vi "Finish Stream.vi"(8 "error in (no error)":errorcluster, 10 "New Mode":T1, 11 "Application in":refnum<class "Application.lvclass">) -> (0 "error out":errorcluster, 3 "Application out":refnum<class "Application.lvclass">)   [LabVIEW 2018, in "Application.lvlib" / "Application.lvclass"]
uses:
  Application.lvclass
  Mode.ctl
  Application.lvclass/Application.ctl
  Hardware/Synchronization Device Messages/Set Streaming Msg/Set Streaming Msg.lvclass/Set Streaming Msg.ctl
  <vilib>/ActorFramework/Message Enqueuer/Message Enqueuer.lvclass/Message Enqueuer.ctl
  Hardware/Tiff Writer/Tiff Writer Messages/Save Tiff Msg/Save Tiff Msg.lvclass/Save Tiff Msg.ctl
  <vilib>/ActorFramework/Message Enqueuer/Enqueue.vi
  Hardware/Synchronization Device Messages/Set Streaming Msg/Set Streaming Msg.lvclass
  C:/Program Files/National Instruments/LabVIEW 2018/vi.lib/ActorFramework/Message/Message.lvclass
  Hardware/Camera Messages/Finish Stream Msg/Finish Stream Msg.lvclass
  Hardware/Tiff Writer/Tiff Writer Messages/Save Tiff Msg/Save Tiff Msg.lvclass
  Resources/GLOBAL/GLOBAL Time-critical.vi
  <vilib>/ActorFramework/Message Priority Queue/Priority Enqueue.vi
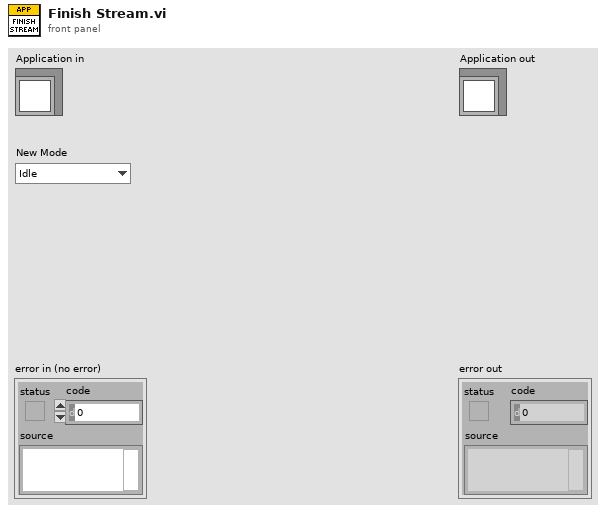
[diagram p1: front panel]
types:
  T1 = typedef "Mode.ctl" = enum16{"Idle", "Cancel", "Live", "Stream", "Autofocus", "Z-Stack"}
  T2 = typedef "Camera Settings.ctl" = cluster{"Exposure Time (ms)":dbl, "Binning":enum16{"1x1", "2x2", "4x4"}, "Scan Mode":i32, "Frames to Acquire":dbl, "Pixel Correction":bool, "Frames to Skip":u32, "File Path":path, "Duty cycle":dbl, "ALEX":bool, "Shutter Enable":bool[], "Timelapse Interval (s)":u32, "fluidics trigger frame":u16}
  T3 = cluster{"Number of Frames":u32, "Image Width (px)":u32, "Image Height (px)":u32, "Pixel Size (nm)":dbl, "Exposure Time (ms)":dbl, "Frame Time (ms)":dbl, "Number of Channels":u32, "Camera Type":enum16{"<unknown>", "Evolve 512", "Orca-Flash 4.0 V2"}, "Bit Depth":u32, "Image Description":string}
  T4 = typedef "Physical Camera Assignment.ctl" = cluster{"Channel Name":string, "Camera Type":T5, "Serial Number":string, "Flip Vertically":bool, "Flip Horizontally":bool, "photonsPerCount":dbl, "wavelength":i16}
  T5 = typedef "Camera Type.ctl" = enum16{"Hamamatsu"}
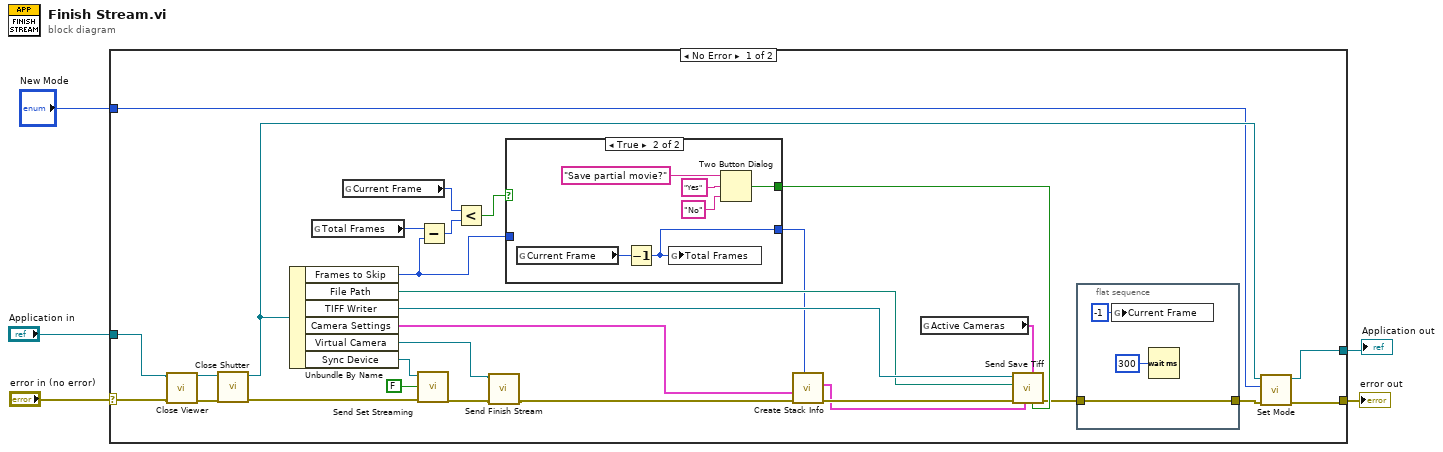
[diagram p0: block diagram]
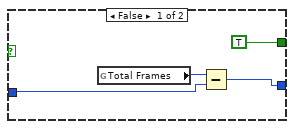
[diagram p2: hidden frame]
diagram:
  n1 = case shown="No Error" "error in (no error)" {
    selector: "error in (no error)" -> [w15 w49]
    tunnel: [w14 w49] -> w4
    tunnel: [w13 w48] -> w2
    tunnel: "Application in" -> [w16 w48]
    tunnel: "New Mode" -> [w9 _]
    frame No Error {
      n2 = call-dynamic "Close Viewer.vi"("error in (no error)"=w15, "Application in"=w16) -> ("error out"=w18:errorcluster, "Application out"=w17:refnum<class "Application.lvclass">)  [unwired: 8 in]
      n3 = call-dynamic "Close Shutter.vi"("error in (no error)"=w18, "Application in"=w17) -> ("error out"=w33:errorcluster, "Application out"=w12:refnum<class "Application.lvclass">)  [unwired: 8 in]
      n4 = Unbundle By Name(w12) -> ("Frames to Skip"=w28:u32, "File Path"=w24:path, "TIFF Writer"=w26:refnum<class "Message Enqueuer.lvclass">, "Camera Settings"=w21:T2, "Virtual Camera"=w6:refnum<class "Message Enqueuer.lvclass">, "Sync Device"=w19:refnum<class "Message Enqueuer.lvclass">)
      n5 = global read "GLOBAL Time-critical.vi" "Total Frames"() -> (w30:i32)
      n6 = global read "GLOBAL Time-critical.vi" "Current Frame"() -> (w31:i32)
      n7 = call "Send Set Streaming.vi"("error in (no error)"=w33, "Streaming?"=FALSE, "Message Enqueuer"=w19) -> ("error out"=w7:errorcluster)  [unwired: 7 in, 1 out]
      n8 = Subtract(x=w30, y=w28) -> (x-y=w29:u32)
      n9 = Less?(x=w31, y=w29) -> (x < y?=w32:bool)
      n10 = call "Send Finish Stream.vi"("error in (no error)"=w7, "Message Enqueuer"=w6) -> ("error out"=w8:errorcluster)  [unwired: 8 in, 1 out]
      n11 = case shown="True" w32 {
        tunnel: [TRUE ("T button?") w44] -> w25
        tunnel: [w38 w43] -> w23
        tunnel: w28 -> [w39 _]
        frame False {
          n12 = global read "GLOBAL Time-critical.vi" "Total Frames"() -> (w40:i32)
          n13 = Subtract(x=w40, y=w39) -> (x-y=w38:u32)
        }
        frame True {
          n14 = global read "GLOBAL Time-critical.vi" "Current Frame"() -> (w42:i32)
          n15 = Decrement(x=w42) -> (x-1=w43:i32)
          n16 = global write "GLOBAL Time-critical.vi" "Total Frames"(w43) -> ()
          n17 = Two Button Dialog(message="Save partial movie?", 1:"No" ("F button name (\"Cancel\")"), 2:"Yes" ("T button name (\"OK\")")) -> (T button?=w44:bool)
        }
      }
      n18 = call "Create Stack Info.vi"("nFrames"=w23, "error in (no error)"=w8, "Camera Settings"=w21) -> ("error out"=w22:errorcluster, "Stack Info"=w20:T3)  [unwired: 7 in]
      n19 = global read "GLOBAL Time-critical.vi" "Active Cameras"() -> (w27:T4[])
      n20 = call "Send Save Tiff.vi"("Cancelled"=w25, "Active Cameras"=w27, "Stack Info"=w20, "error in (no error)"=w22, "File Path"=w24, "Message Enqueuer"=w26) -> ("error out"=w10:errorcluster)  [unwired: 4 in, 1 out]
      n21 = flat-sequence {
        tunnel: [w37] -> w11
        tunnel: w10 -> [w37]
        frame #0 {
          n22 = global write "GLOBAL Time-critical.vi" "Current Frame"(-1 ("Current Frame")) -> ()
          n23 = Wait (ms)(milliseconds to wait=u32 300) -> ()  [unwired: 1 out]
        }
      }
      n24 = call-dynamic "Set Mode.vi"("error in (no error)"=w11, "New Mode"=w9, "Application in"=w12) -> ("error out"=w14:errorcluster, "Application out"=w13:refnum<class "Application.lvclass">)  [unwired: 7 in]
    }
    frame Error {
    }
  }
  "error out" <- w4
  "Application out" <- w2
